vi "Global.vi"() -> ()   [LabVIEW 2018]
panel:
  in  "C8":bool
  in  "C7":bool
  in  "C6":bool
  in  "C5":bool
  in  "C4":bool
  in  "C3":bool
  in  "C2":bool
  in  "C1":bool
  in  "B8":bool
  in  "B7":bool
  in  "B6":bool
  in  "B5":bool
  in  "B4":bool
  in  "B3":bool
  in  "B2":bool
  in  "B1":bool
  in  "A8":bool
  in  "A7":bool
  in  "A6":bool
  in  "A5":bool
  in  "A4":bool
  in  "A3":bool
  in  "A2":bool
  in  "A1":bool
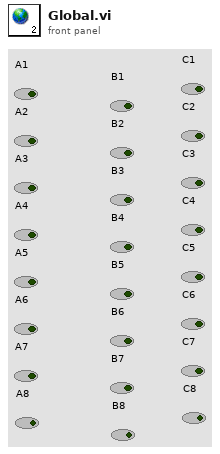
[diagram p1: front panel]
diagram:
